vi "DCAM_acquire_n_frames_to_dcimg.vi"() -> ()   [LabVIEW 2015]
panel:
  in  "Start Button":bool
  out "Frames Recorded":i32
  in  "Frames":i32=100
  in  "stop":bool
  out "Image":u16[][](graph)
  out "error out":errorcluster
  out "Timeseries save path":path
  out "Timeseries Base Filename":string
  out "Model":string
  out "Camera ID":string
  out "Firmware":string
  out "DCAM Ver.":string
  out "Library Ver.":string
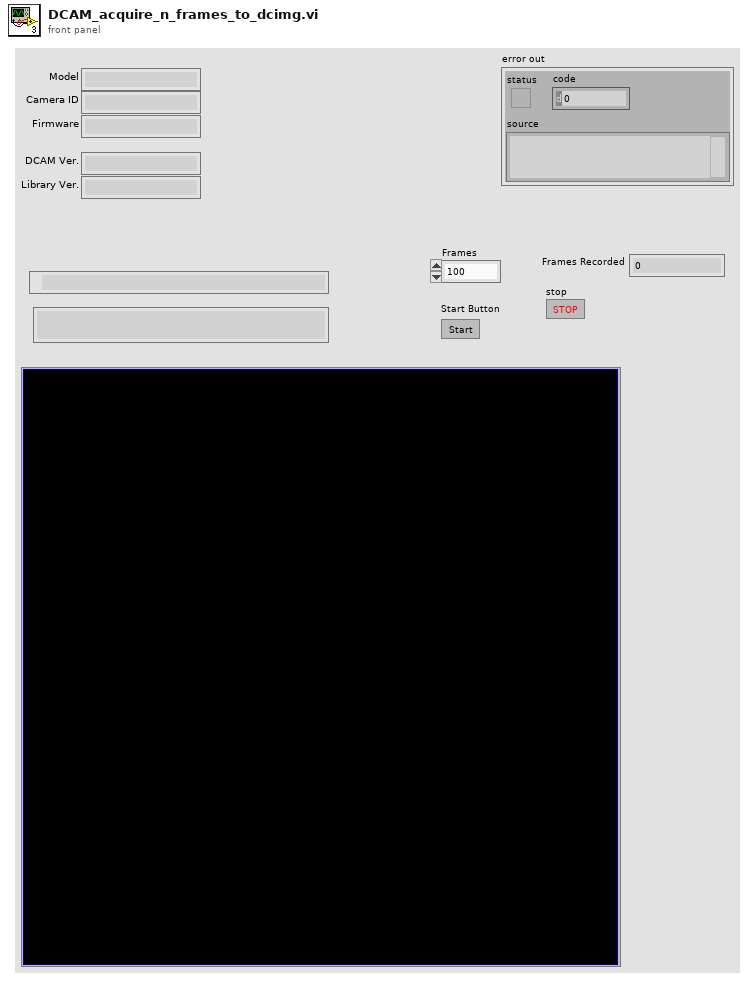
[diagram p1: front panel]
types:
  T1 = cluster{"Capture Library":string, "DCAM-API":string}
  T2 = cluster{"Model":string, "Camera ID":string, "Firmware":string}
  T3 = cluster{"height":u32, "width":u32, "datatype":u32}
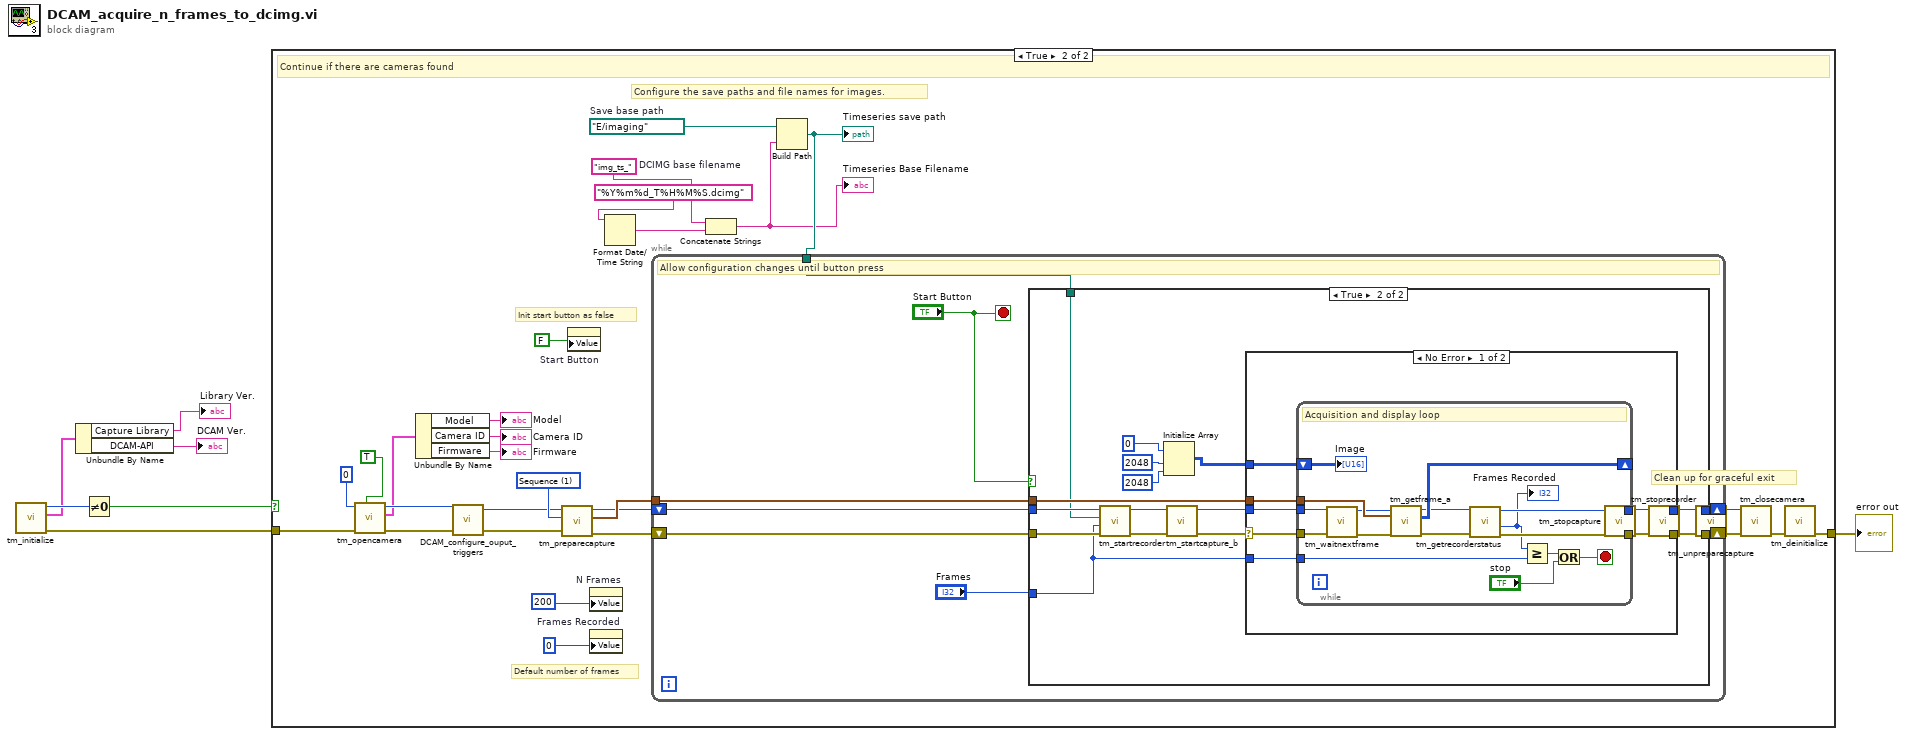
[diagram p0: block diagram]
diagram:
  n1 = call <userlib>:"tm_initialize.vi"() -> ("error out"=w2:errorcluster, "Version Info"=w5:T1, "Number Of Cameras"=w7:u32)  [unwired: 8 in, 1 out]
  n2 = Unbundle By Name(w5) -> ("Capture Library"=→"Library Ver.":string, "DCAM-API"=→"DCAM Ver.":string)
  n3 = Not Equal To 0?(x=w7) -> (x != 0?=w6:bool)
  n4 = case shown="True" w6 {
    tunnel: w2 -> [w8 w41]
    tunnel: [w8 w30] -> w1
    frame False {
    }
    frame True {
      w29 = 1 items=["Snap", "Sequence"] ("Capture mode")
      w13 = "img_ts_"  # DCIMG base filename
      w16 = path "E:/imaging"  # Save base path
      # "Init start button as false"
      # "Clean up for graceful exit"
      # "Default number of frames"
      # "Configure the save paths and file names for images."
      # "Continue if there are cameras found"
      n5 = call <userlib>:"tm_opencamera.vi"("Force Open"=TRUE, "error in (no error)"=w41, "Camera Index"=0) -> ("error out"=w38:errorcluster, "Camera Details"=w34:T2, "Handle out"=w39:u32)  [unwired: 6 in]
      n6 = Unbundle By Name(w34) -> ("Model"=→"Model":string, "Camera ID"=→"Camera ID":string, "Firmware"=→"Firmware":string)
      n7 = call "DCAM_configure_ouput_triggers.vi"("error in (no error)"=w38, "Handle in"=w39) -> ("error out"=w28:errorcluster, "Handle out"=w27:u32)  [unwired: 2 in]
      n8 = call <userlib>:"tm_preparecapture.vi"("error in (no error)"=w28, "Capture mode"=w29, "Handle in"=w27) -> ("error out"=w24:errorcluster, "Buffer Info"=w26:T3, "Handle out"=w25:u32)  [unwired: 5 in, 1 out]
      n9 = property on="Start Button" class="Bool (strict)"("Value"=FALSE) -> ()  [unwired: 2 in, 2 out]
      n10 = property on="N Frames" class="DigNum (strict)"("Value"=200) -> ()  [unwired: 2 in, 2 out]
      n11 = property on="Frames Recorded" class="DigNum (strict)"("Value"=0) -> ()  [unwired: 2 in, 2 out]
      n12 = Format Date/Time String(time format string (%c)="%Y%m%d_T%H%M%S.dcimg" ("name or relative path")) -> (date/time string=w14:string)  [unwired: 2 in]
      n13 = Concatenate Strings(w13, w14) -> (w11:string)
      "Timeseries Base Filename" <- w11
      n14 = Build Path(base path=w16, name or relative path=w11) -> (appended path=w12:path)
      "Timeseries save path" <- w12
      n15 = while {
        tunnel: w26 -> [w50]
        tunnel: w12 -> [w45]
        shift-right: [w47] -> w22
        shift-left: w25 -> [w49]
        shift-right: [w46] -> w21
        shift-left: w24 -> [w48]
        stop <- "Start Button" stop-if-true
        # "Allow configuration changes until button press"
        n16 = case shown="True" "Start Button" {
          tunnel: w50 -> [_ w67]
          tunnel: w49 -> [w52 w59]
          tunnel: w48 -> [w51 w58]
          tunnel: [w52 w57] -> w47
          tunnel: [w51 w56] -> w46
          tunnel: "Frames" -> [_ w55]
          tunnel: w45 -> [_ w53]
          frame False {
          }
          frame True {
            n17 = call <userlib>:"tm_startrecorder.vi"("error in (no error)"=w58, "frames"=w55, "File"=w53, "Handle in"=w59) -> ("error out"=w61:errorcluster, "Handle out"=w60:u32)  [unwired: 6 in]
            n18 = Initialize Array(u16 0 ("element"), 2048 ("dimension size"), 2048 ("dimension size")) -> (w62:u16[][])
            n19 = call <userlib>:"tm_startcapture_b.vi"("error in (no error)"=w61, "Handle in"=w60) -> ("error out"=w54:errorcluster, "Handle out"=w66:u32)  [unwired: 8 in]
            n20 = case shown="No Error" w54 {
              selector: w54 -> [w68 w92]
              tunnel: w67 -> [w74 _]
              tunnel: w66 -> [w73 w91]
              tunnel: w62 -> [w72 _]
              tunnel: [w71 w91] -> w57
              tunnel: [w70 w92] -> w56
              tunnel: w55 -> [w69 _]
              frame No Error {
                n21 = while {
                  tunnel: w74 -> [w90]
                  tunnel: w73 -> [w89]
                  tunnel: w68 -> [w86]
                  shift-right: [w84] -> _
                  shift-left: w72 -> [w85]
                  tunnel: [w81] -> w71
                  tunnel: [w80] -> w70
                  tunnel: w69 -> [w75]
                  stop <- w78 stop-if-true
                  # "Acquisition and display loop"
                  n22 = call <userlib>:"tm_waitnextframe.vi"("error in (no error)"=w86, "Handle in"=w89) -> ("error out"=w87:errorcluster, "Handle out"=w88:u32)  [unwired: 6 in, 2 out]
                  n23 = call <userlib>:"tm_getframe_a.vi"("error in (no error)"=w87, "Buffer Info"=w90, "Handle in"=w88) -> ("error out"=w83:errorcluster, "Data 16"=w84:u16[][], "Handle out"=w82:u32)  [unwired: 4 in, 2 out]
                  n24 = call <userlib>:"tm_getrecorderstatus.vi"("error in (no error)"=w83, "Handle"=w82) -> ("error out"=w80:errorcluster, "Count"=w76:i32, "Handle"=w81:u32)  [unwired: 6 in, 1 out]
                  "Frames Recorded" <- w76
                  n25 = Greater Or Equal?(x=w76, y=w75) -> (x >= y?=w77:bool)
                  n26 = Or(x=w77, y="stop") -> (x .or. y?=w78:bool)
                  "Image" <- w85
                }
              }
              frame Error {
              }
            }
          }
        }
      }
      n27 = call <userlib>:"tm_stopcapture.vi"("error in (no error)"=w21, "Handle in"=w22) -> ("error out"=w17:errorcluster, "Handle out"=w18:u32)  [unwired: 8 in]
      n28 = call <userlib>:"tm_stoprecorder.vi"("error in (no error)"=w17, "Handle in"=w18) -> ("error out"=w19:errorcluster, "Handle out"=w20:u32)  [unwired: 8 in]
      n29 = call <userlib>:"tm_unpreparecapture.vi"("error in (no error)"=w19, "Handle in"=w20) -> ("error out"=w33:errorcluster, "Handle out"=w32:u32)  [unwired: 8 in]
      n30 = call <userlib>:"tm_closecamera.vi"("error in (no error)"=w33, "Handle in"=w32) -> ("error out"=w31:errorcluster)  [unwired: 9 in]
      n31 = call <userlib>:"tm_deinitialize.vi"("error in (no error)"=w31) -> ("error out"=w30:errorcluster)  [unwired: 10 in]
    }
  }
  "error out" <- w1
